vi "Engine Out - Faults - Fuel Pressure.vi"(11 "Fuel Pressure [kPa]":sgl) -> ()   [LabVIEW 2015, in "ECS-RT.lvlib"]
uses:
  ECS-RT.lvlib
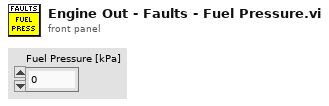
[diagram p1: front panel]
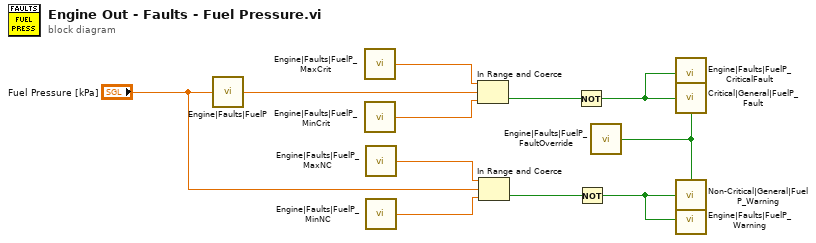
[diagram p0: block diagram]
diagram:
  n1 = call "Engine|Faults|FuelP"("Value"="Fuel Pressure [kPa]") -> ()
  n2 = call "Engine|Faults|FuelP_MaxCrit"() -> ("Value"=w5:sgl)
  n3 = call "Engine|Faults|FuelP_MinCrit"() -> ("Value"=w4:sgl)
  n4 = call "Engine|Faults|FuelP_MaxNC"() -> ("Value"=w9:sgl)
  n5 = call "Engine|Faults|FuelP_MinNC"() -> ("Value"=w8:sgl)
  n6 = In Range and Coerce(upper limit=w5, x="Fuel Pressure [kPa]", lower limit=w4) -> (In Range?=w3:bool)  [unwired: 1 out]
  n7 = In Range and Coerce(upper limit=w9, x="Fuel Pressure [kPa]", lower limit=w8) -> (In Range?=w7:bool)  [unwired: 1 out]
  n8 = Not(x=w3) -> (.not. x?=w6:bool)
  n9 = Not(x=w7) -> (.not. x?=w10:bool)
  n10 = call "Engine|Faults|FuelP_FaultOverride"() -> ("Value"=w1:bool)
  n11 = call "Engine|Faults|FuelP_CriticalFault"("Value"=w6) -> ()
  n12 = call "Critical|General|FuelP_Fault"("Fault"=w6, "Override (F)"=w1) -> ()  [unwired: 1 in]
  n13 = call "Non-Critical|General|FuelP_Warning"("Fault"=w10, "Override (F)"=w1) -> ()  [unwired: 1 in]
  n14 = call "Engine|Faults|FuelP_Warning"("Value"=w10) -> ()
